vi "ScaleSingleWaveformGEECS.vi"(10 "waveform info in":T1, 11 "I16 in":i16[](array[numeric])) -> (2 "waveform info out":T2, 3 "Waveform":waveform(dbl))   [LabVIEW 2013, in "Tektronix MDO MSO DPO.lvclass"]
uses:
  Tektronix MDO MSO DPO.lvclass
  Waveform_attributes.ctl
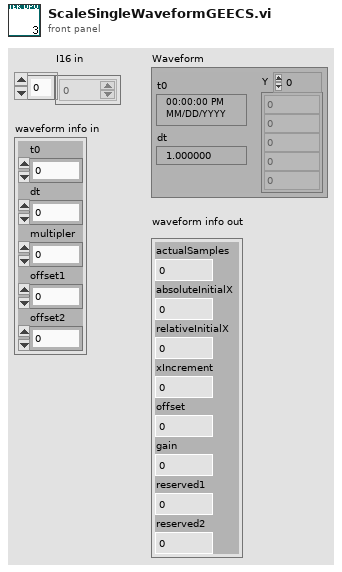
[diagram p1: front panel]
types:
  T1 = typedef "Waveform_attributes.ctl" = cluster{"t0":dbl, "dt":dbl, "multipler":dbl, "offset1":dbl, "offset2":dbl}
  T2 = cluster{"actualSamples":i32, "absoluteInitialX":dbl, "relativeInitialX":dbl, "xIncrement":dbl, "offset":dbl, "gain":dbl, "reserved1":dbl, "reserved2":dbl}
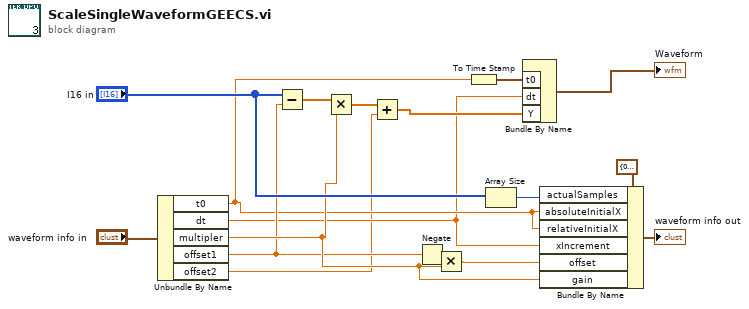
[diagram p0: block diagram]
diagram:
  n1 = Unbundle By Name("waveform info in") -> ("t0"=w9:dbl, "dt"=w7:dbl, "multipler"=w15:dbl, "offset1"=w12:dbl, "offset2"=w5:dbl)
  n2 = Subtract(x="I16 in", y=w12) -> (x-y=w4:dbl[])
  n3 = Multiply(x=w4, y=w15) -> (x*y=w3:dbl[])
  n4 = Add(x=w3, y=w5) -> (x+y=w16:dbl[])
  n5 = Negate(x=w12) -> (-x=w13:dbl)
  n6 = Multiply(x=w13, y=w15) -> (x*y=w14:dbl)
  n7 = To Time Stamp(1:w9) -> (0:w2:timestamp)
  n8 = Array Size(array="I16 in") -> (size(s)=w8:i32)
  n9 = Bundle By Name("t0"=w2, "dt"=w7, "Y"=w16) -> (→"Waveform":waveform(dbl))  [unwired: 1 in]
  n10 = Bundle By Name(cluster=T2 {"actualSamples"=0, "absoluteInitialX"=0.0, "relativeInitialX"=0.0, "xIncrement"=0.0, "offset"=0.0, "gain"=0.0, "reserved1"=0.0, "reserved2"=0.0} ("waveform info"), "actualSamples"=w8, "absoluteInitialX"=w9, "relativeInitialX"=w9, "xIncrement"=w7, "offset"=w14, "gain"=w15) -> (→"waveform info out":T2)
